vi "_A33LoadArbitraryVolat.vi"(1 "WFM (Column) Number":i32, 2 "Array WFM":i16[](array[numeric]), 4 "Timeout (40000 ms)":u32=40000, 5 "WFM Source":u16(ring) items=["Single file", "Split files", "Array"], 6 "WFM Length":i32, 7 "ARB Number":u32=1, 8 "error in (no error)":errorcluster, 9 "WFM Path":path, 10 "Channel (1: Channel1)":u16(ring)=1 items=["Channel1"=1, "Channel2"=2], 11 "VISA resource name":refnum<visa-resource-name>) -> (0 "error out":errorcluster, 3 "VISA resource name out":refnum<visa-resource-name>)   [LabVIEW 2012]
doc: "Creates and saves an arbitrary waveform in edit memory. \n\n<B>Note:</B>\n\nCreates an arbitrary waveform in edit memory and because of this, the waveform will remain stored on the instrument until deleted. If any sensitive information is contained in the arbitrary waveform, it is recommended that the waveform be deleted when finished."
uses:
  <vilib>/Utility/file.llb/Read From Spreadsheet File (I64).vi
panel:
  out "Attempts":i32
  # "Load waveform into arb\nmemory of a certain channel\nunder name 'ARB#'\nIf WFM alerady exists - use ClearArbitrary\n4M points in total per channel"
  # "No dots in the file name!"
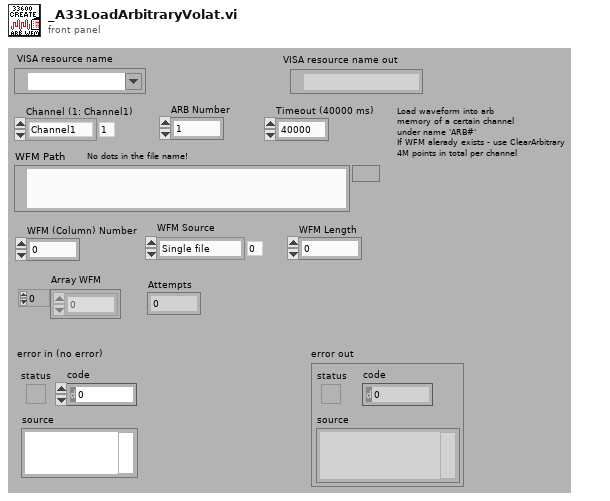
[diagram p1: front panel]
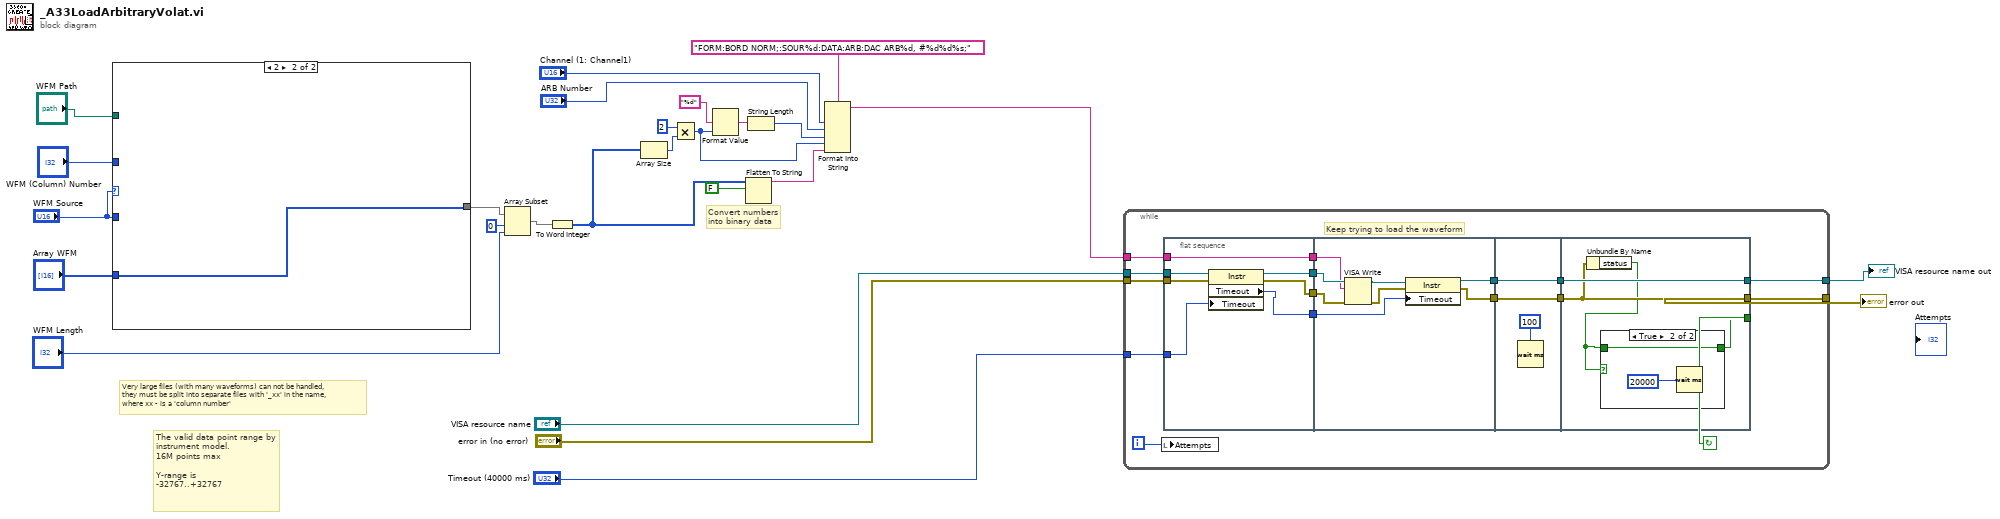
[diagram p0: block diagram]
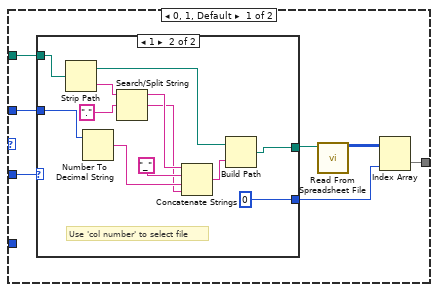
[diagram p2: hidden frame]
diagram:
  # "Very large files (with many waveforms) can not be handled,\nthey must be split into separate files with '_xx' in the name,\nwhere xx - is a 'column number'"
  # "Convert numbers\ninto binary data"
  # "The valid data point range by instrument model. \n16M points max\n\nY-range is\n-32767..+32767"
  n1 = case shown="2" "WFM Source" {
    tunnel: [w32 w48] -> w26
    tunnel: "WFM Path" -> [w31 _]
    tunnel: "WFM (Column) Number" -> [w30 _]
    tunnel: "WFM Source" -> [w27 _]
    tunnel: "Array WFM" -> [_ w48]
    frame 0, 1, Default {
      n2 = case shown="1" w27 {
        tunnel: w31 -> [w35 w47]
        tunnel: w30 -> [w34 w44]
        tunnel: [w35 w37] -> w29
        tunnel: [w34 0 ("x")] -> w28
        frame 0, Default {
          # "File contains multiple wfms"
        }
        frame 1 {
          # "Use 'col number' to select file"
          n3 = Strip Path(path=w47) -> (stripped path=w39:path, name=w45:string)
          n4 = Number To Decimal String(number=w44) -> (decimal integer string=w41:string)  [unwired: 1 in]
          n5 = Search/Split String(string=w45, search string/char (-)=".") -> (substring before match=w43:string, match + rest of string=w40:string)  [unwired: 1 in, 1 out]
          n6 = Concatenate Strings(w43, "_", w41, w40) -> (w38:string)
          n7 = Build Path(base path=w39, name or relative path=w38) -> (appended path=w37:path)
        }
      }
      n8 = call-poly <vilib>:"Read From Spreadsheet File.vi"("file path (dialog if empty)"=w29) -> ("all rows"=w33:i64[][])  [unwired: 6 in, 4 out]
      n9 = Index Array(array=w33, index (col)=w28) -> (element=w32:i64[])  [unwired: 1 in]
    }
    frame 2 {
    }
  }
  n10 = Array Subset(array=w26, index=0 ("x"), length="WFM Length") -> (w16:i64[])
  n11 = To Word Integer(number=w16) -> (16bit integer=w17:i16[])
  n12 = Array Size(array=w17) -> (size(s)=w23:i32)
  n13 = Multiply(x=2, y=w23) -> (x*y=w6:i32)
  n14 = Format Value(format string="%d", value (0)=w6) -> (output string=w20:string)  [unwired: 1 in]
  n15 = Flatten To String(anything=w17, prepend array or string size? (T)=FALSE) -> (data string=w5:string)  [unwired: 2 in, 2 out]
  n16 = String Length(string=w20) -> (length=w7:i32)
  n17 = Format Into String(format string="FORM:BORD NORM;:SOUR%d:DATA:ARB:DAC ARB%d, #%d%d%s;" ("string"), "Channel (1: Channel1)", "ARB Number", w7, w6, w5) -> (resulting string=w4:string)  [unwired: 2 in, 1 out]
  n18 = while {
    tunnel: w4 -> [w60]
    tunnel: "Timeout (40000 ms)" -> [w59]
    tunnel: "VISA resource name" -> [w58]
    tunnel: "error in (no error)" -> [w57]
    tunnel: [w56] -> w12
    tunnel: [w55] -> w11
    i -> [w53]
    stop <- w54 continue-if-true
    # "Keep trying to load the waveform"
    n19 = local write "Attempts"(w53) -> ()
    n20 = flat-sequence {
      tunnel: [w71] -> w64
      tunnel: [w70] -> w63
      tunnel: [w69] -> w62
      tunnel: w60 -> [w68]
      tunnel: [w68] -> w61
      tunnel: w59 -> [w67]
      tunnel: w58 -> [w66]
      tunnel: w57 -> [w65]
      tunnel: w64 -> [w75]
      tunnel: w63 -> [w76]
      tunnel: w62 -> [w77]
      tunnel: w61 -> [w74]
      tunnel: [w73] -> w52
      tunnel: [w72] -> w50
      tunnel: w52 -> [w82]
      tunnel: [w82] -> w51
      tunnel: w50 -> [w81]
      tunnel: [w81] -> w49
      tunnel: [w86] -> w55
      tunnel: [w85] -> w56
      tunnel: w51 -> [w85]
      tunnel: w49 -> [w86]
      tunnel: [w83] -> w54
      frame #0 {
        n21 = property class="Instr"(reference=w66, error in=w65, "Timeout"=w67) -> (reference out=w71:refnum<visa-resource-name>, error out=w70:errorcluster, "Timeout"=w69:u32)
      }
      frame #1 {
        n22 = VISA Write(VISA resource name=w75, write buffer=w74, error in (no error)=w76) -> (VISA resource name out=w78:refnum<visa-resource-name>, error out=w79:errorcluster)  [unwired: 1 out]
        n23 = property class="Instr"(reference=w78, error in=w79, "Timeout"=w77) -> (reference out=w72:refnum<visa-resource-name>, error out=w73:errorcluster)
      }
      frame #2 {
        n24 = Wait (ms)(milliseconds to wait=100 ("x")) -> ()  [unwired: 1 out]
      }
      frame #3 {
        n25 = Unbundle By Name(w85) -> ("status"=w84:bool)
        n26 = case shown="True" w84 {
          tunnel: w84 -> [w87 w88]
          tunnel: [w87 w88] -> w83
          frame False {
          }
          frame True {
            n27 = Wait (ms)(milliseconds to wait=20000 ("x")) -> ()  [unwired: 1 out]
          }
        }
      }
    }
  }
  "error out" <- w12
  "VISA resource name out" <- w11
